vi "Read.vi"(8 "error in (no error)":errorcluster, 11 "Current Time in":refnum<class "Const_Current Time.lvclass">) -> (0 "error out":errorcluster, 2 "Time Stamp":timestamp, 3 "Current Time out":refnum<class "Const_Current Time.lvclass">)   [LabVIEW 2021, in "Const_Current Time.lvclass"]
uses:
  Const_Current Time.lvclass
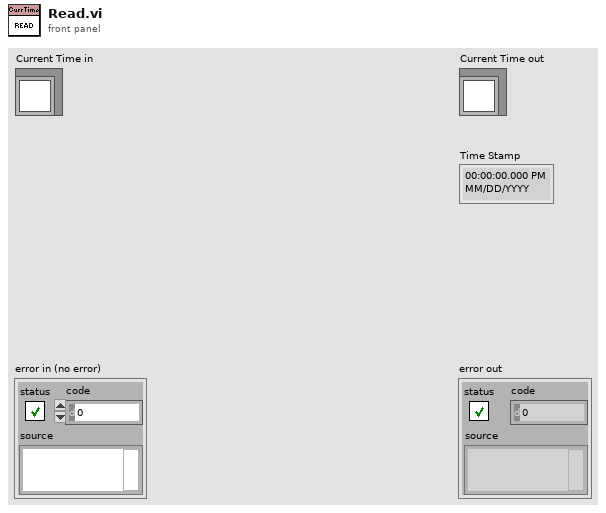
[diagram p1: front panel]
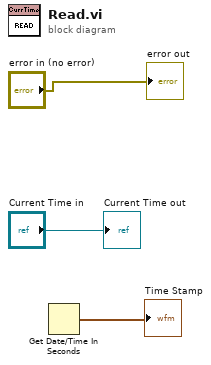
[diagram p0: block diagram]
diagram:
  n1 = Get Date/Time In Seconds() -> (seconds since 1Jan1904=→"Time Stamp":timestamp)
  "error out" <- "error in (no error)"
  "Current Time out" <- "Current Time in"
